vi "UTIL Get Timestamp.vi"() -> (1 "current time":timestamp, 3 "appended array":dbl[](array[numeric]))   [LabVIEW 2017]
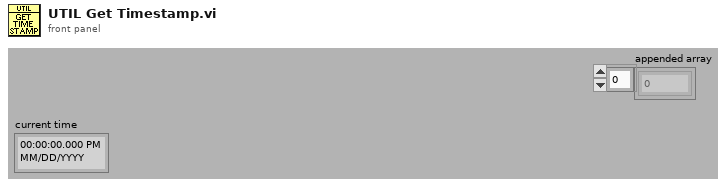
[diagram p1: front panel]
types:
  T1 = typedef "LVDateTimeRec.ctl" = cluster{"fractional second":dbl, "second":i32, "minute":i32, "hour":i32, "day of month":i32, "month":i32, "year":i32, "day of week":i32, "day of year":i32, "DST":i32}
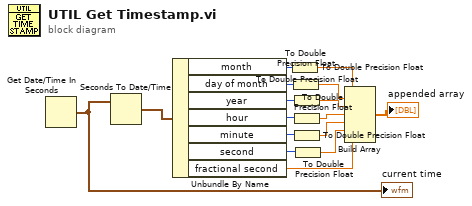
[diagram p0: block diagram]
diagram:
  n1 = Get Date/Time In Seconds() -> (seconds since 1Jan1904=w9:timestamp)
  "current time" <- w9
  n2 = Seconds To Date/Time(time stamp (now)=w9) -> (date time rec=w10:T1)  [unwired: 1 in]
  n3 = Unbundle By Name(w10) -> ("month"=w11:i32, "day of month"=w12:i32, "year"=w13:i32, "hour"=w14:i32, "minute"=w15:i32, "second"=w16:i32, "fractional second"=w1:dbl)
  n4 = To Double Precision Float(number=w11) -> (double precision float=w5:dbl)
  n5 = To Double Precision Float(number=w12) -> (double precision float=w4:dbl)
  n6 = To Double Precision Float(number=w13) -> (double precision float=w6:dbl)
  n7 = To Double Precision Float(number=w14) -> (double precision float=w7:dbl)
  n8 = To Double Precision Float(number=w15) -> (double precision float=w8:dbl)
  n9 = To Double Precision Float(number=w16) -> (double precision float=w2:dbl)
  n10 = Build Array(w5, w4, w6, w7, w8, w2, w1) -> (→"appended array":dbl[])
